vi "Condition Select.vi"(8 "error in (no error)":T2, 11 "array in":string[][](array[string])) -> (0 "error out":T2, 1 "OK?":bool, 2 "Panel Close?":bool, 3 "Array":T1[](array[typedef]))   [LabVIEW 2018]
uses:
  CTL/Tags.ctl
panel:
  out "Anchor Fore":bool
  out "Mast Fore":bool
  out "Manuvering Light":bool
  out "Stern":bool
  out "Mast Aft":bool
  out "Anchor Aft":bool
  out "Side Light  Port":bool
  out "Side Light STBD":bool
  in  "Cancel":bool
  in  "OK":bool
  in  "Select Condition":i32(listbox)
  # "SELECT CONDITION"
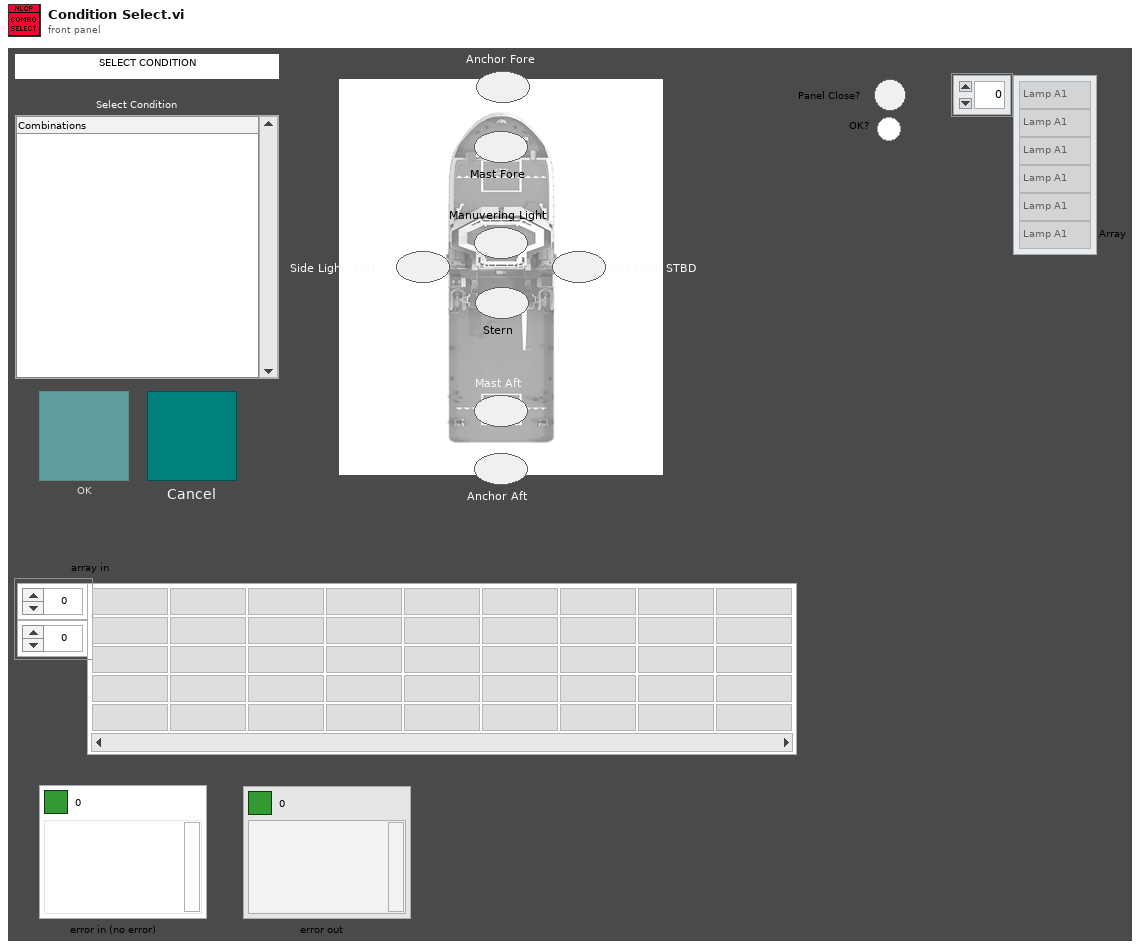
[diagram p1: front panel]
types:
  T1 = typedef "Tags.ctl" = enum16{"Lamp A1", "Lamp B1", "Lamp C1", "Lamp D1", "Lamp E1", "Lamp F1", "Lamp G1", "Lamp H1", "Lamp A2", "Lamp B2", "Lamp C2", "Lamp D2", "Lamp E2", "Lamp F2", "Lamp G2", "Lamp H2", "Ack A1", "Ack B1", "Ack C1", "Ack D1", "Ack E1", "Ack F1", "Ack G1", "Ack H1", "Ack A2", "Ack B2", "Ack C2", "Ack D2", "Ack E2", "Ack F2", "Ack G2", "Ack H2", "SSM", "SAS", "LSM", ""}
  T2 = cluster{"Boolean Round":bool, "code":i32, "source":string}
  T3 = enum32{"Invalid", "Standard", "Closed", "Hidden", "Minimized", "Maximized"}
  T4 = enum8{"Enabled", "Disabled", "Disabled and Grayed Out"}
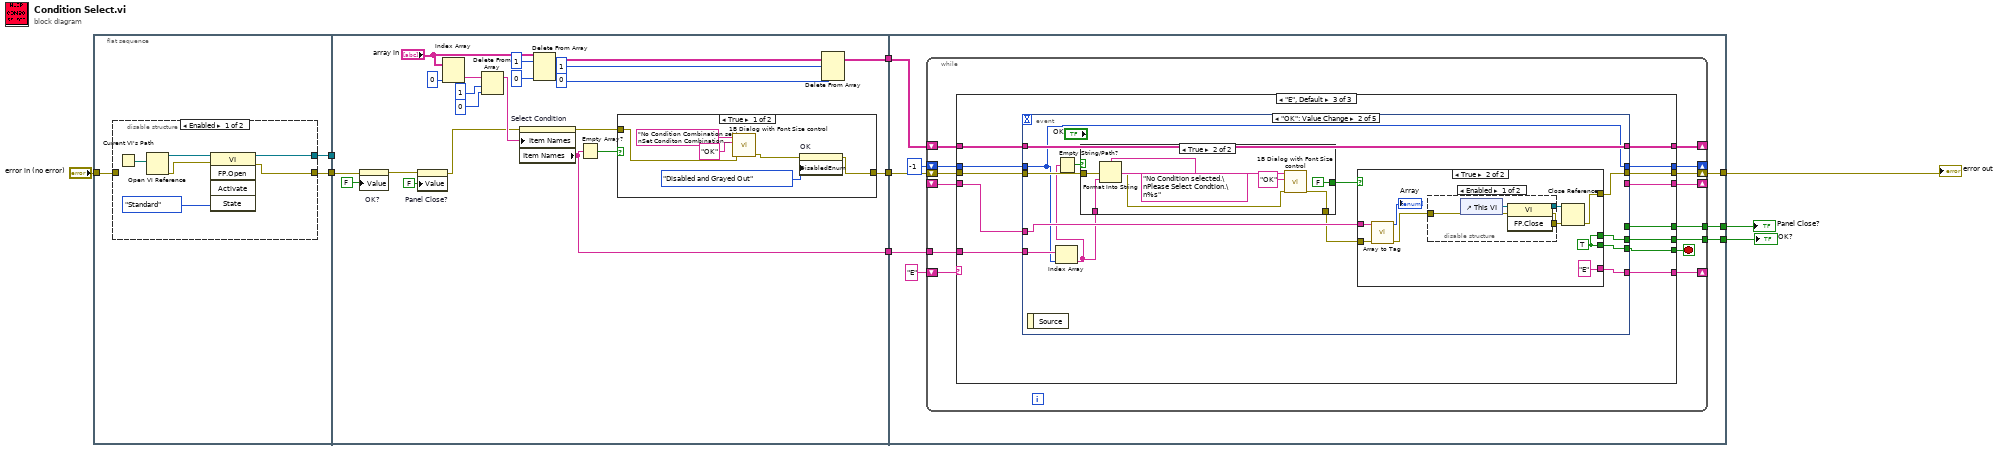
[diagram p0: block diagram]
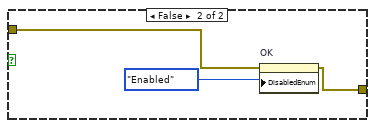
[diagram p3: hidden frame]
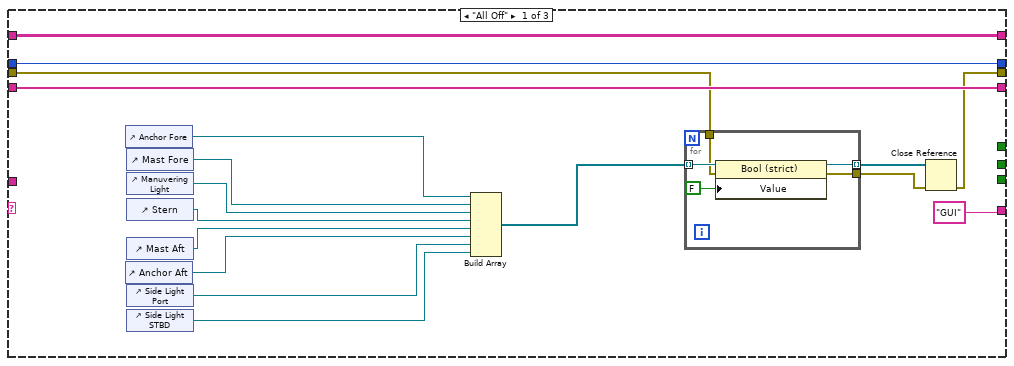
[diagram p4: hidden frame]
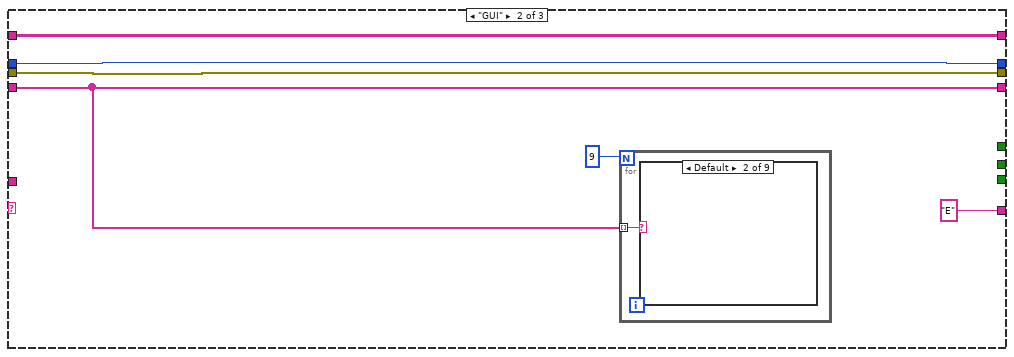
[diagram p5: hidden frame]
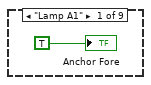
[diagram p6: hidden frame]
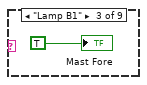
[diagram p7: hidden frame]
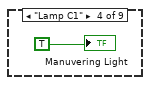
[diagram p8: hidden frame]
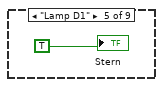
[diagram p9: hidden frame]
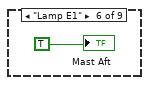
[diagram p10: hidden frame]
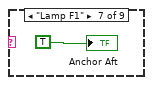
[diagram p11: hidden frame]
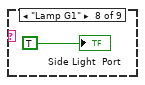
[diagram p12: hidden frame]
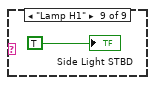
[diagram p13: hidden frame]
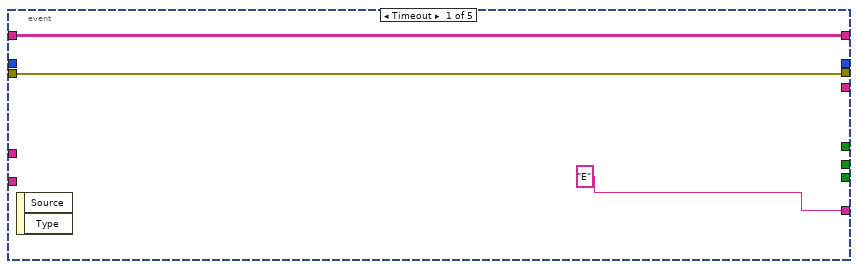
[diagram p14: hidden frame]
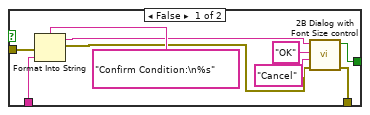
[diagram p15: hidden frame]
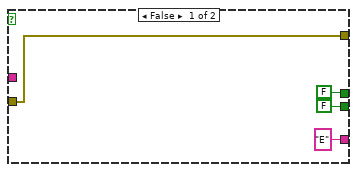
[diagram p16: hidden frame]
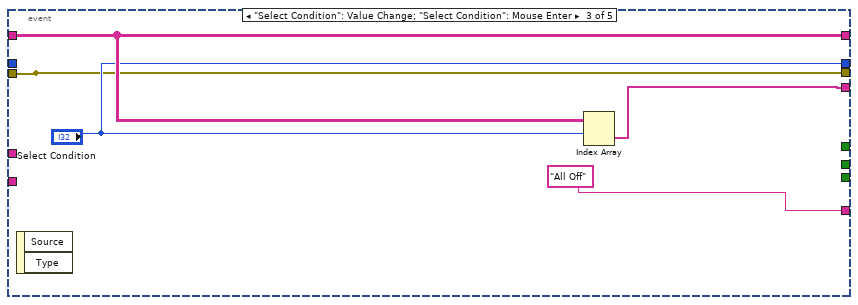
[diagram p18: hidden frame]
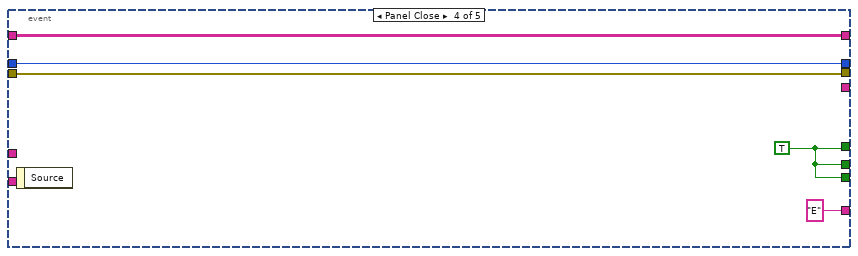
[diagram p19: hidden frame]
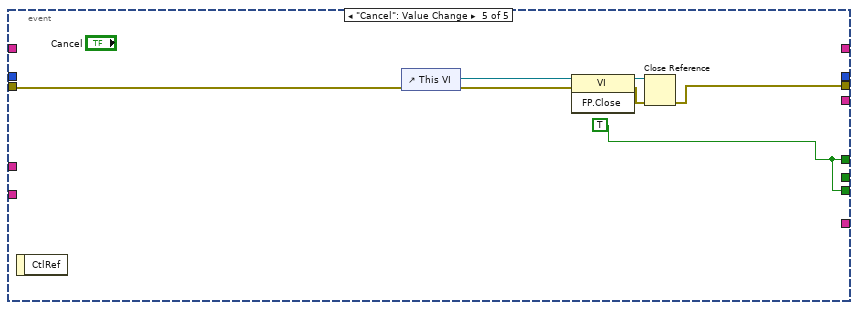
[diagram p20: hidden frame]
diagram:
  n1 = flat-sequence {
    tunnel: [w12] -> w9
    tunnel: [w11] -> w7
    tunnel: "error in (no error)" -> [w10]
    tunnel: w9 -> [w29]
    tunnel: [w26] -> w8
    tunnel: w7 -> [_]
    tunnel: [w21] -> w2
    tunnel: [w20] -> w1
    tunnel: w8 -> [w56]
    tunnel: [w57] -> w4
    tunnel: [w55] -> w5
    tunnel: [w53] -> w3
    tunnel: w2 -> [w52]
    tunnel: w1 -> [w50]
    frame #0 {
      n2 = disable-structure shown="Enabled" {
        disable-tunnel: [w14 w19] -> w12
        disable-tunnel: [w13 _] -> w11
        disable-tunnel: w10 -> [_ w19]
        frame Enabled {
          n3 = Current VI's Path() -> (path=w18:path)
          n4 = Open VI Reference(vi path=w18) -> (vi reference=w17:refnum<vi>, error out=w16:errorcluster)  [unwired: 5 in]
          n5 = invoke class="VI" method="FP.Open"(reference=w17, error in=w16, "State"=T3."Standard") -> (reference out=w13:refnum<vi>, error out=w14:errorcluster)  [unwired: 2 in, 3 out]
        }
        frame Disabled {
        }
      }
    }
    frame #1 {
      n6 = property on="OK?" class="Bool (strict)"(error in=w29, "Value"=FALSE ("OK?")) -> (error out=w30:errorcluster)  [unwired: 1 in, 1 out]
      n7 = property on="Panel Close?" class="Bool (strict)"(error in=w30, "Value"=FALSE ("Panel Close?")) -> (error out=w31:errorcluster)  [unwired: 1 in, 1 out]
      n8 = Index Array(array="array in", index (col)=0 ("disabled index (col)")) -> (element=w39:string[])  [unwired: 1 in]
      n9 = Delete From Array(array=w39, length=1, index=0) -> (array with subset deleted=w33:string[])  [unwired: 1 out]
      n10 = property on="Select Condition" class="LstBox (strict)"(error in=w31, "Item Names"=w33) -> (error out=w22:errorcluster, "Item Names"=w20:string[])  [unwired: 1 in, 1 out]
      n11 = Delete From Array(array="array in", length=1, index (col)=0 ("disabled index (col)")) -> (array with subset deleted=w27:string[][])  [unwired: 1 in, 1 out]
      n12 = Empty Array?(array=w20) -> (empty?=w23:bool)
      n13 = case shown="True" w23 {
        tunnel: w22 -> [w42 w48]
        tunnel: [w45 w47] -> w21
        frame True {
          n14 = call "1B Dialog with Font Size control.vi"("error in (no error)"=w42, "T Button Name (\"OK\")"="OK" ("button name (\"OK\")"), "message"="No Condition Combination set.\nSet Conditon Combination using configure button.") -> ("error out"=w41:errorcluster)  [unwired: 7 in, 1 out]
          n15 = property on="OK" class="Bool"(error in=w41, "DisabledEnum"=T4."Disabled and Grayed Out" ("Disabled")) -> (error out=w45:errorcluster)  [unwired: 1 in, 1 out]
        }
        frame False {
          n16 = property on="OK" class="Bool"(error in=w48, "DisabledEnum"=T4."Enabled" ("Disabled")) -> (error out=w47:errorcluster)  [unwired: 1 in, 1 out]
        }
      }
      n17 = Delete From Array(array=w27, length=1, index (row)=0) -> (array with subset deleted=w26:string[][])  [unwired: 1 in, 1 out]
    }
    frame #2 {
      n18 = while {
        shift-right: [w70] -> w57
        shift-left: w52 -> [w71]
        tunnel: [w67] -> w55
        shift-right: [w64] -> _
        shift-left: w56 -> [w69]
        shift-right: [w65] -> _
        shift-left: "E" -> [w66]
        shift-right: [w63] -> _
        shift-left: -1 ("Select Condition") -> [w62]
        shift-right: [w61] -> _
        shift-left: _ -> [w60]
        tunnel: [w59] -> w53
        tunnel: w50 -> [w58]
        stop <- w68 stop-if-true
        n19 = case shown="\"E\", Default" w66 {
          tunnel: w71 -> [w74 w98 w121]
          tunnel: [w73 w98 w110] -> w70
          tunnel: w69 -> [w88 w96 w120]
          tunnel: [_ _ w119] -> w68
          tunnel: [_ _ w118] -> w67
          tunnel: ["GUI" "E" w117] -> w65
          tunnel: [w88 w96 w116] -> w64
          tunnel: [w87 w97 w115] -> w63
          tunnel: w62 -> [w87 w97 w113]
          tunnel: [w86 w95 w114] -> w61
          tunnel: w60 -> [w86 w95 w111]
          tunnel: [_ _ w112] -> w59
          tunnel: w58 -> [_ _ w109]
          frame "All Off" {
            n20 = control-ref of="Anchor Fore"() -> (w84:refnum<vi>)
            n21 = control-ref of="Anchor Aft"() -> (w79:refnum<vi>)
            n22 = control-ref of="Mast Fore"() -> (w83:refnum<vi>)
            n23 = control-ref of="Manuvering Light"() -> (w82:refnum<vi>)
            n24 = control-ref of="Stern"() -> (w81:refnum<vi>)
            n25 = control-ref of="Mast Aft"() -> (w80:refnum<vi>)
            n26 = control-ref of="Side Light  Port"() -> (w78:refnum<vi>)
            n27 = control-ref of="Side Light STBD"() -> (w77:refnum<vi>)
            n28 = Build Array(w84, w83, w82, w81, w80, w79, w78, w77) -> (w85:refnum<vi>[])
            n29 = for {
              tunnel: [w92] -> w75
              tunnel: [w91] -> w76 mode=indexing
              tunnel: w85 -> [w90] mode=indexing
              tunnel: w74 -> [w89]
              n30 = property class="Bool (strict)"(reference=w90, error in=w89, "Value"=FALSE) -> (reference out=w91:refnum<vi>, error out=w92:errorcluster)
            }
            n31 = Close Reference(reference=w76, error in (no error)=w75) -> (error out=w73:errorcluster)
          }
          frame "GUI" {
            n32 = for {
              N: 9 -> [_]
              tunnel: w95 -> [w100] mode=indexing
              n33 = case shown="Default" w100 {
                frame "Lamp A1" {
                  "Anchor Fore" <- TRUE ("Anchor Fore")
                }
                frame Default {
                }
                frame "Lamp B1" {
                  "Mast Fore" <- TRUE ("Mast Fore")
                }
                frame "Lamp C1" {
                  "Manuvering Light" <- TRUE ("Manuvering Light")
                }
                frame "Lamp D1" {
                  "Stern" <- TRUE ("Stern")
                }
                frame "Lamp E1" {
                  "Mast Aft" <- TRUE ("Mast Aft")
                }
                frame "Lamp F1" {
                  "Anchor Aft" <- TRUE ("Anchor Aft")
                }
                frame "Lamp G1" {
                  "Side Light  Port" <- TRUE ("Side Light  Port")
                }
                frame "Lamp H1" {
                  "Side Light STBD" <- TRUE ("Side Light STBD")
                }
              }
            }
          }
          frame "E", Default {
            n34 = event shown="[1] \"OK\": Value Change" {
              selector: _ -> [_ _ _ _ _]
              dyn-events: _ -> [_ _ _ _ _]
              timeout: _ -> [_ _ _ _ _]
              tunnel: w121 -> [w124 w137 w172 w180 w183]
              tunnel: [w124 w133 w172 w180 w182] -> w110
              tunnel: w120 -> [w123 w131 w175 w181 _]
              tunnel: [_ w134 _ w177 w187] -> w119
              tunnel: [_ _ _ w177 w187] -> w118
              tunnel: ["E" w136 "All Off" "E" _] -> w117
              tunnel: [w123 w131 w175 w181 _] -> w116
              tunnel: [_ w125 "Select Condition" w178 _] -> w115
              tunnel: [_ _ w173 _ _] -> w114
              tunnel: w113 -> [_ w125 _ w178 _]
              tunnel: [_ w135 _ w177 _] -> w112
              tunnel: w111 -> [_ w132 _ _ _]
              tunnel: [_ _ w172 _ _] -> _
              tunnel: w109 -> [_ w130 _ _ _]
              event Timeout {
                n35 = event-data() -> ()  [unwired: 1 in, 2 out]
              }
              event "OK": Value Change {
                n36 = event-data() -> ()  [unwired: 1 in, 1 out]
                n37 = Index Array(array=w130, index=w125) -> (element=w128:string)
                n38 = Empty String/Path?(string/path=w128) -> (empty?=w129:bool)
                n39 = case shown="True" w129 {
                  tunnel: w137 -> [w146 w154]
                  tunnel: w128 -> [w144 w152]
                  tunnel: [w140 w147] -> w127
                  tunnel: [w139 FALSE ("OK")] -> w126
                  frame False {
                    n40 = Format Into String(format string="Confirm Condition:\n%s", error in=w146, w144) -> (resulting string=w138:string, error out=w141:errorcluster)  [unwired: 1 in]
                    n41 = call "2B Dialog with Font Size control.vi"("error in (no error)"=w141, "F Button Name (\"Cancel\")"="Cancel" ("F Button Name (\"Cancel\")"), "T Button Name (\"OK\")"="OK" ("T Button Name (\"OK\")"), "message"=w138) -> ("error out"=w140:errorcluster, "OK"=w139:bool)  [unwired: 6 in]
                  }
                  frame True {
                    n42 = Format Into String(format string="No Condition selected.\nPlease Select Condtion.\n%s", error in=w154, w152) -> (resulting string=w149:string, error out=w148:errorcluster)  [unwired: 1 in]
                    n43 = call "1B Dialog with Font Size control.vi"("error in (no error)"=w148, "T Button Name (\"OK\")"="OK" ("button name (\"OK\")"), "message"=w149) -> ("error out"=w147:errorcluster)  [unwired: 7 in, 1 out]
                  }
                }
                n44 = case shown="True" w126 {
                  tunnel: ["E" "E"] -> w136
                  tunnel: [FALSE w166] -> w135
                  tunnel: [FALSE w166] -> w134
                  tunnel: [w155 w163] -> w133
                  tunnel: w132 -> [_ w162]
                  tunnel: w127 -> [w155 w159]
                  frame False {
                  }
                  frame True {
                    w166 = TRUE
                    n45 = call "Array to Tag.vi"("error in (no error)"=w159, "1D array"=w162) -> ("error out"=w160:T2, "Array"=→"Array":T1[])  [unwired: 8 in]
                    n46 = disable-structure shown="Enabled" {
                      disable-tunnel: [w170 _] -> w165
                      disable-tunnel: [w169 _] -> w164
                      disable-tunnel: w160 -> [w168 _]
                      frame Enabled {
                        n47 = control-ref of="This VI"() -> (w171:refnum<vi>)
                        n48 = invoke class="VI" method="FP.Close"(reference=w171, error in=w168) -> (reference out=w169:refnum<vi>, error out=w170:errorcluster)  [unwired: 1 in, 1 out]
                      }
                      frame Disabled {
                      }
                    }
                    n49 = Close Reference(reference=w164, error in (no error)=w165) -> (error out=w163:errorcluster)
                  }
                }
              }
              event "Select Condition": Value Change; "Select Condition": Mouse Enter {
                n50 = event-data() -> ()  [unwired: 1 in, 2 out]
                n51 = Index Array(array=w175, index (row)="Select Condition") -> (element=w173:string[])  [unwired: 1 in]
              }
              event Panel Close {
                w177 = TRUE
                n52 = event-data() -> ()  [unwired: 1 in, 1 out]
              }
              event "Cancel": Value Change {
                w187 = TRUE
                n53 = event-data() -> ()  [unwired: 1 in, 1 out]
                n54 = control-ref of="This VI"() -> (w186:refnum<vi>)
                n55 = invoke class="VI" method="FP.Close"(reference=w186, error in=w183) -> (reference out=w184:refnum<vi>, error out=w185:errorcluster)  [unwired: 1 in, 1 out]
                n56 = Close Reference(reference=w184, error in (no error)=w185) -> (error out=w182:errorcluster)
              }
            }
          }
        }
      }
    }
  }
  "error out" <- w4
  "Panel Close?" <- w5
  "OK?" <- w3
